vi "ROVPingWrite.vi"(8 "error in (no error)":errorcluster, 11 "VISA Refnum in":refnum<visa-resource-name>) -> (0 "error out":errorcluster, 3 "VISA Refnum out":refnum<visa-resource-name>)   [LabVIEW 2019]
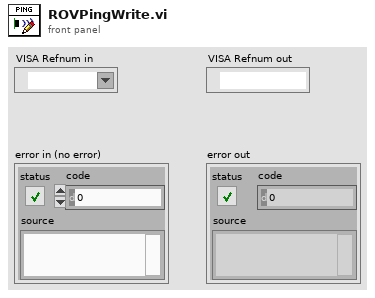
[diagram p1: front panel]
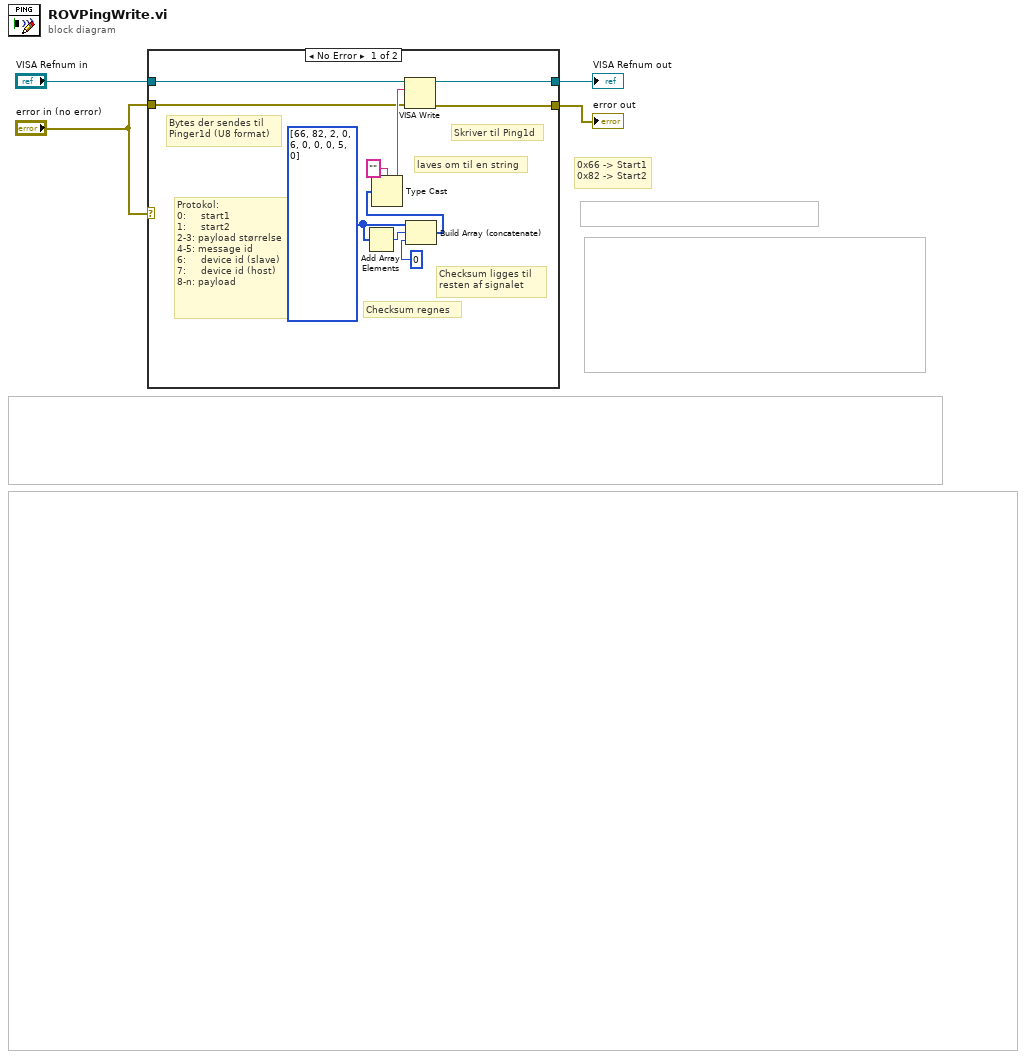
[diagram p0: block diagram]
diagram:
  # "0x66 -> Start1\n0x82 -> Start2"
  n1 = case shown="No Error" "error in (no error)" {
    tunnel: [w14 w16] -> w4
    tunnel: [w13 w15] -> w3
    tunnel: "VISA Refnum in" -> [w6 w15]
    tunnel: "error in (no error)" -> [w5 w16]
    frame No Error {
      w7 = u8[] [66, 82, 2, 0, 6, 0, 0, 0, 5, 0]
      # "Protokol:\n0:     start1\n1:     start2\n2-3: payload størrelse\n4-5: message id\n6:     device id (slave)\n7:     device id (host)\n8-n: payload"
      # "Bytes der sendes til\nPinger1d (U8 format)"
      # "Skriver til Ping1d"
      # "laves om til en string"
      # "Checksum regnes"
      # "Checksum ligges til \nresten af signalet"
      n2 = Add Array Elements(numeric array=w7) -> (sum=w8:u8)
      n3 = Build Array (concatenate)(w7, w8, u8 0 ("element")) -> (w10:u8[])
      n4 = Type Cast(type="", x=w10) -> (*(type *) &x=w12:string)
      n5 = VISA Write(VISA resource name=w6, write buffer=w12, error in (no error)=w5) -> (VISA resource name out=w13:refnum<visa-resource-name>, error out=w14:errorcluster)  [unwired: 1 out]
    }
    frame Error {
    }
  }
  "error out" <- w4
  "VISA Refnum out" <- w3
